vi "Read.vi"(8 "error in (no error)":errorcluster, 11 "Stop Seq Command Config in":refnum<class "Stop Seq Command Config.lvclass">) -> (0 "error out":errorcluster, 2 "Sequence":string, 3 "Stop Seq Command Config out":refnum<class "Stop Seq Command Config.lvclass">)   [LabVIEW 2020, in "VolatusSeqConfig.lvlib" / "Stop Seq Command Config.lvclass"]
uses:
  Stop Seq Command Config.lvclass
  Stop Seq Command Config.lvclass/Stop Seq Command Config.ctl
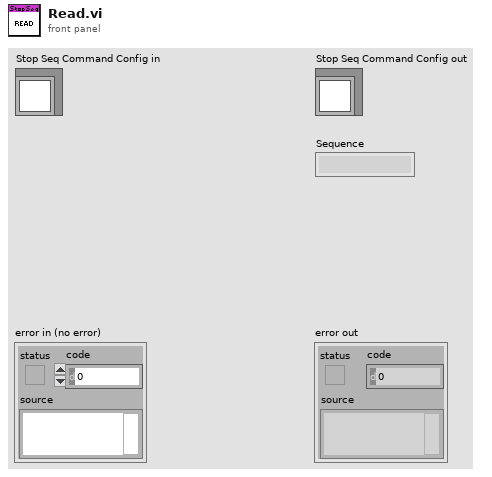
[diagram p1: front panel]
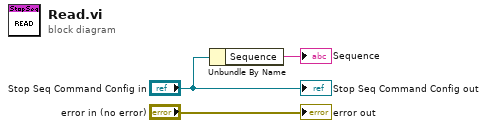
[diagram p0: block diagram]
diagram:
  n1 = Unbundle By Name("Stop Seq Command Config in") -> ("Sequence"=→"Sequence":string)
  "error out" <- "error in (no error)"
  "Stop Seq Command Config out" <- "Stop Seq Command Config in"
